vi "write_params.vi"(8 "error in (no error)":errorcluster, 10 "params":T1={"penalty"="l2", "loss"="squared_hinge", "dual"=TRUE, "tol"=0.0001, "C"=1.0, "multi_class"="ovr", "fit_intercept"=TRUE, "intercept_scaling"=1.0, "class_weight"={"class_weight_type"="None", "class_weight_dict"="{\"class_label\":1.2}"}, "verbose"=0.0, "random_state"=0.0, "max_iter"=1000.0}, 11 "LinearSVC in":refnum<class "LinearSVC.lvclass">) -> (0 "error out":errorcluster, 3 "LinearSVC out":refnum<class "LinearSVC.lvclass">)   [LabVIEW 2020, in "LinearSVC.lvclass"]
uses:
  LinearSVC.lvclass
  Controls/linear_svc_params.ctl
  LinearSVC.lvclass/LinearSVC.ctl
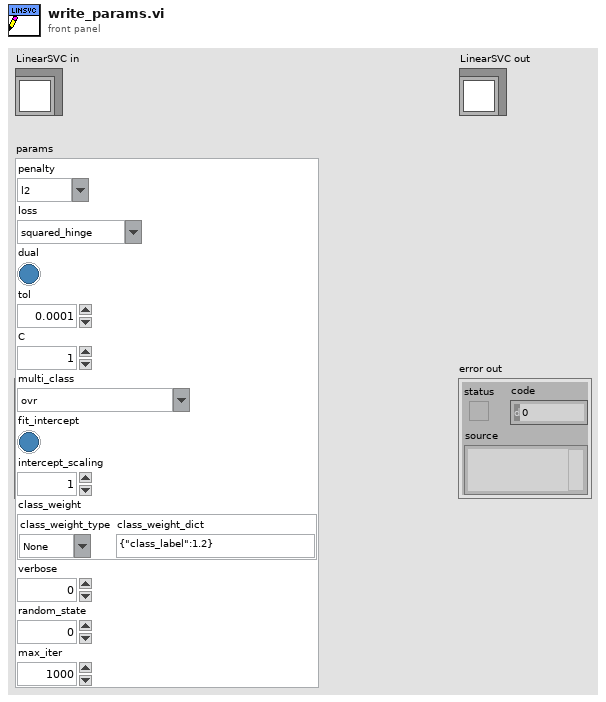
[diagram p1: front panel]
types:
  T1 = typedef "linear_svc_params.ctl" = cluster{"penalty":string, "loss":string, "dual":bool, "tol":dbl, "C":dbl, "multi_class":string, "fit_intercept":bool, "intercept_scaling":dbl, "class_weight":cluster{"class_weight_type":string, "class_weight_dict":string}, "verbose":dbl, "random_state":dbl, "max_iter":dbl}
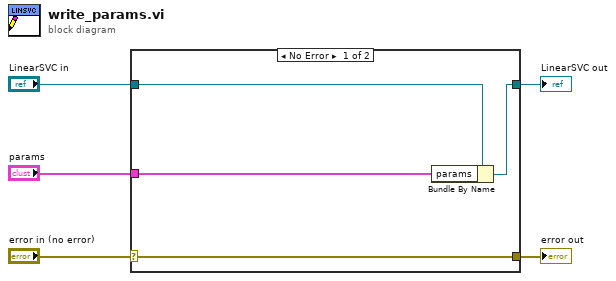
[diagram p0: block diagram]
diagram:
  n1 = case shown="No Error" "error in (no error)" {
    selector: "error in (no error)" -> [w9 w10]
    tunnel: [w9 w10] -> w4
    tunnel: [w7 w11] -> w2
    tunnel: "LinearSVC in" -> [w8 w11]
    tunnel: "params" -> [w6 _]
    frame No Error {
      n2 = Bundle By Name(cluster=w8, "params"=w6) -> (w7:refnum<class "LinearSVC.lvclass">)
    }
    frame Error {
    }
  }
  "error out" <- w4
  "LinearSVC out" <- w2
